vi "Channel list header ---constant.vi"() -> (3 "Column Header Strings":string[](array[string])=["Analog inputs", "Analog outputs", "Digital inputs", "Digital outputs", "Counter inputs"])   [LabVIEW 2020, in "NI DAQ.lvlib"]
uses:
  NI DAQ.lvlib
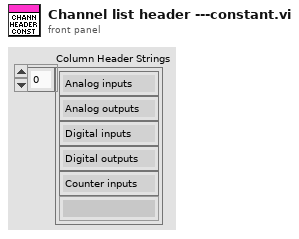
[diagram p1: front panel]
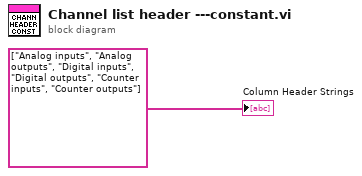
[diagram p0: block diagram]
diagram:
  "Column Header Strings" <- string[] ["Analog inputs", "Analog outputs", "Digital inputs", "Digital outputs", "Counter inputs", "Counter outputs"] ("Column Header Strings[]")
